vi "Read Config File.vi"(8 "error in (no error)":errorcluster, 11 "Config In":refnum<class "Excel_class.lvclass">=refnum) -> (0 "error out":errorcluster, 2 "Calibration Configuration Out":T1, 3 "DAQmx Cluster Out":T2 {"ai DAQmx Cluster"."input terminal configuration" items=["Default"=-1, "RSE"=10083, "NRSE"=10078, "Differential"=10106, "Pseudodifferential"=12529]; "bc DAQmx Cluster"."Scaling Information"."electrical units" items=["Volts/Volt"=15896, "mVolts/Volt"=15897]; "bc DAQmx Cluster"."Scaling Information"."physical units" items=["Newtons"=15875, "Pounds"=15876, "kgf"=15877]; "bc DAQmx Cluster"."Bridge Information"."bridge configuration" items=["Full Bridge"=10182, "Half Bridge"=10187, "Quarter Bridge"=10270]; "bc DAQmx Cluster"."Bridge Information"."voltage excitation source" items=["Internal"=10200, "External"=10167]; "tc DAQmx Cluster"."Thermocouple Type" items=["J"=10072, "K"=10073, "N"=10077, "R"=10082, "S"=10085, "T"=10086, "B"=10047, "E"=10055]; "tc DAQmx Cluster"."Units" items=["Deg C"=10143, "Deg F"=10144, "Kelvins"=10325, "Deg R"=10145, "From Custom Scale"=10065]})   [LabVIEW 2024]
uses:
  Calibration Configuration.ctl
  DAQmx Configuration.ctl
  <vilib>/ATEsystem/CLAUDIE_xlsx/Excel_class/Excel_class.lvclass
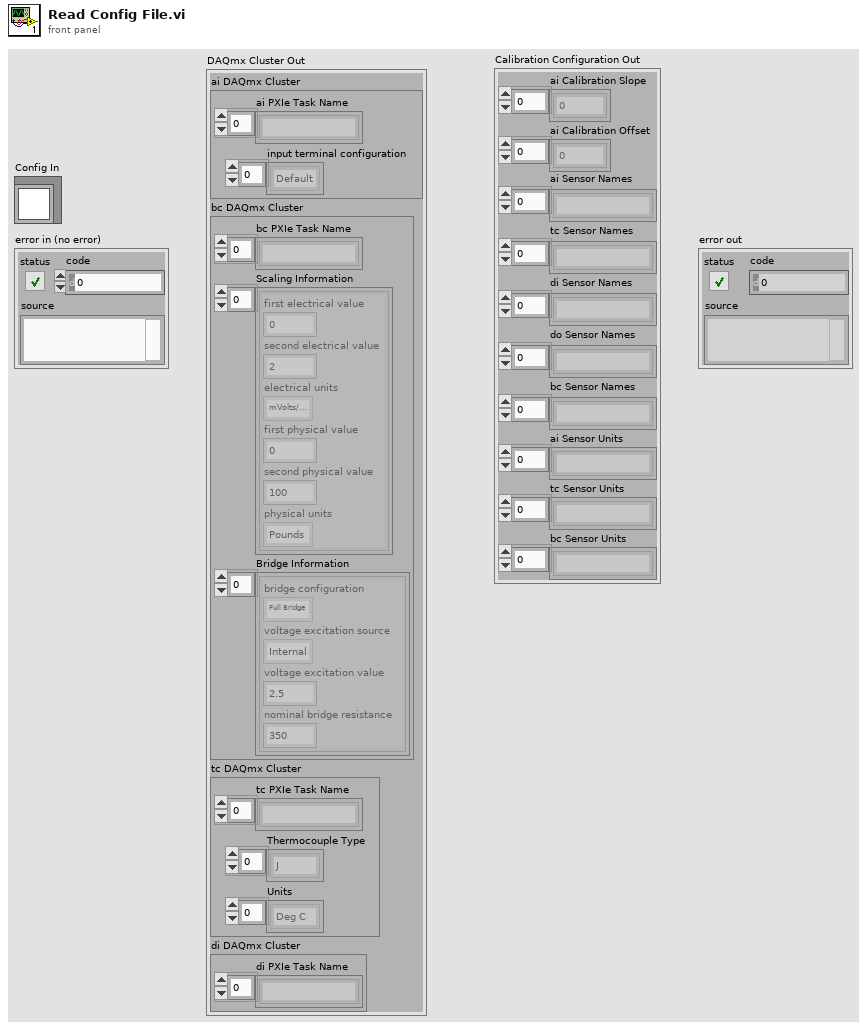
[diagram p1: front panel]
types:
  T1 = typedef "Calibration Configuration.ctl" = cluster{"ai Calibration Slope":dbl[], "ai Calibration Offset":dbl[], "ai Sensor Names ":string[], "tc Sensor Names":string[], "di Sensor Names":string[], "do Sensor Names":string[], "bc Sensor Names":string[], "ai Sensor Units":string[], "tc Sensor Units":string[], "bc Sensor Units":string[]}
  T2 = typedef "DAQmx Configuration.ctl" = cluster{"ai DAQmx Cluster":cluster{"ai PXIe Task Name":string[], "input terminal configuration":i32[]}, "bc DAQmx Cluster":cluster{"bc PXIe Task Name":string[], "Scaling Information":cluster{"first electrical value":dbl, "second electrical value":dbl, "electrical units":i32, "first physical value":dbl, "second physical value":dbl, "physical units":i32}[], "Bridge Information":cluster{"bridge configuration":i32, "voltage excitation source":i32, "voltage excitation value":dbl, "nominal bridge resistance":dbl}[]}, "tc DAQmx Cluster":cluster{"tc PXIe Task Name":string[], "Thermocouple Type":i32[], "Units":i32[]}, "di DAQmx Cluster":cluster{"di PXIe Task Name":string[]}}
  T3 = cluster{"ai PXIe Task Name":string[], "input terminal configuration":i32[]}
  T4 = cluster{"bc PXIe Task Name":string[], "Scaling Information":cluster{"first electrical value":dbl, "second electrical value":dbl, "electrical units":i32, "first physical value":dbl, "second physical value":dbl, "physical units":i32}[], "Bridge Information":cluster{"bridge configuration":i32, "voltage excitation source":i32, "voltage excitation value":dbl, "nominal bridge resistance":dbl}[]}
  T5 = cluster{"tc PXIe Task Name":string[], "Thermocouple Type":i32[], "Units":i32[]}
  T6 = cluster{dbl, dbl, "electrical units":i32, dbl, dbl, "physical units":i32}
  T7 = cluster{"bridge configuration":i32, "voltage excitation source":i32, dbl, dbl}
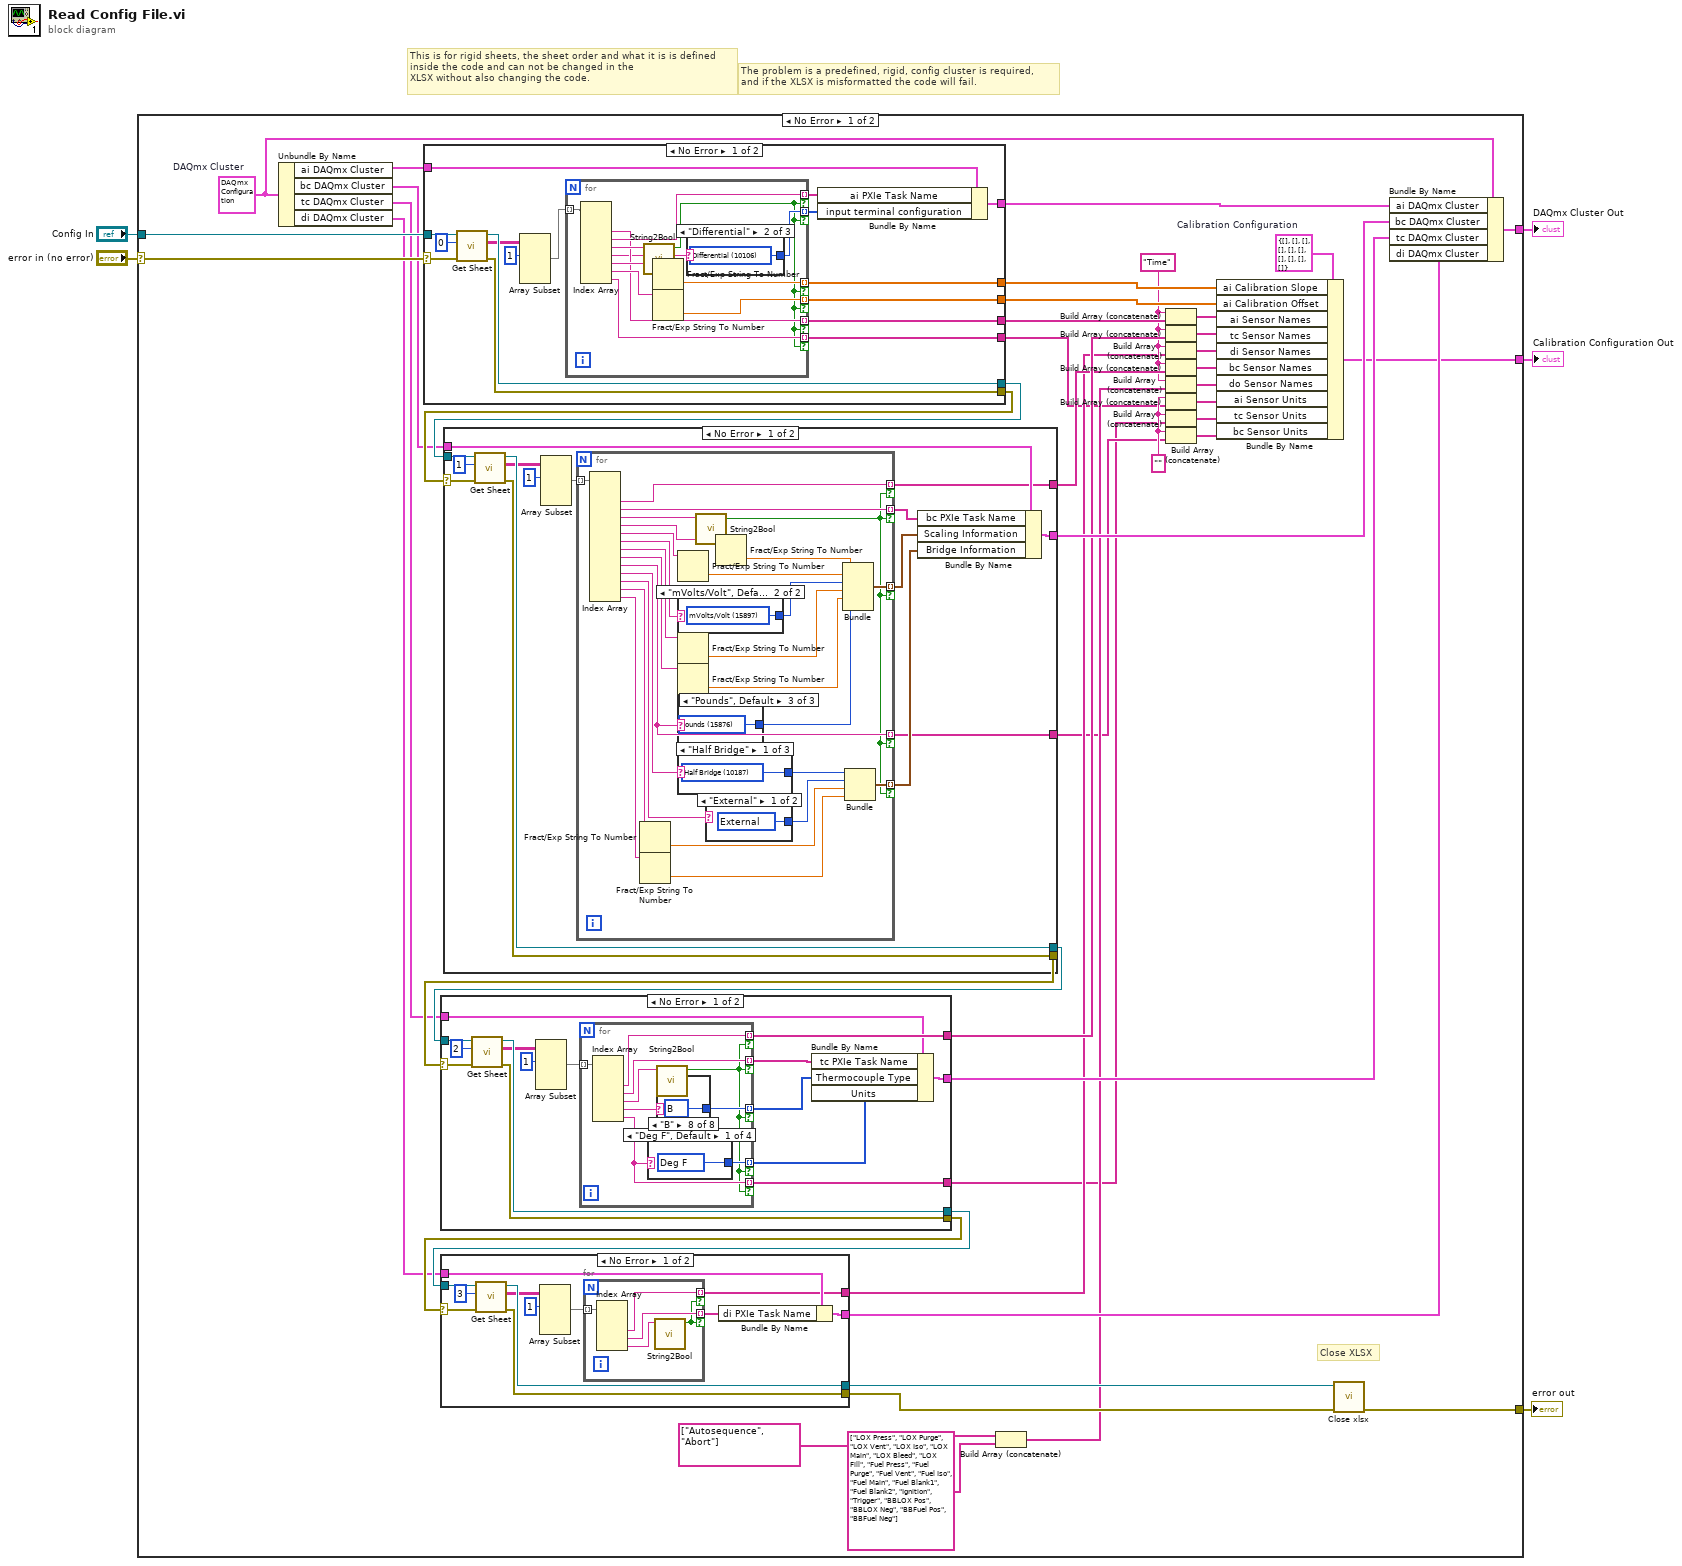
[diagram p0: block diagram]
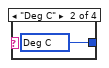
[diagram p3: hidden frame]
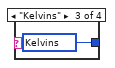
[diagram p4: hidden frame]
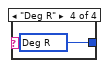
[diagram p5: hidden frame]
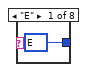
[diagram p6: hidden frame]
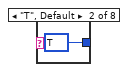
[diagram p7: hidden frame]
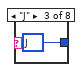
[diagram p8: hidden frame]
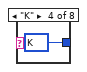
[diagram p9: hidden frame]
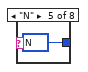
[diagram p10: hidden frame]
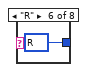
[diagram p11: hidden frame]
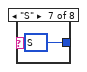
[diagram p12: hidden frame]
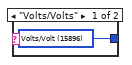
[diagram p14: hidden frame]
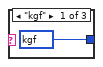
[diagram p15: hidden frame]
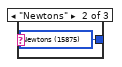
[diagram p16: hidden frame]
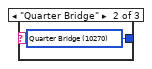
[diagram p17: hidden frame]
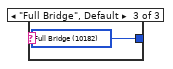
[diagram p18: hidden frame]
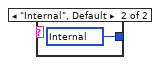
[diagram p19: hidden frame]
diagram:
  # "The problem is a predefined, rigid, config cluster is required,\nand if the XLSX is misformatted the code will fail."
  # "This is for rigid sheets, the sheet order and what it is is defined\ninside the code and can not be changed in the\nXLSX without also changing the code."
  n1 = case shown="No Error" "error in (no error)" {
    selector: "error in (no error)" -> [w37 w196]
    tunnel: [w50 w196] -> w4
    tunnel: [w43 _] -> w2
    tunnel: "Config In" -> [w38 _]
    tunnel: [w26 _] -> w1
    frame No Error {
      w11 = ""
      w17 = "Time"
      w32 = T1 {"ai Calibration Slope"=[], "ai Calibration Offset"=[], "ai Sensor Names "=[], "tc Sensor Names"=[], "di Sensor Names"=[], "do Sensor Names"=[], "bc Sensor Names"=[], "ai Sensor Units"=[], "tc Sensor Units"=[], "bc Sensor Units"=[]}  # Calibration Configuration
      w36 = T2 {"ai DAQmx Cluster"={"ai PXIe Task Name"=[], "input terminal configuration"=[]}, "bc DAQmx Cluster"={"bc PXIe Task Name"=[], "Scaling Information"=[], "Bridge Information"=[]}, "tc DAQmx Cluster"={"tc PXIe Task Name"=[], "Thermocouple Type"=[], "Units"=[]}, "di DAQmx Cluster"={"di PXIe Task Name"=[]}}  # DAQmx Cluster
      # "Close XLSX"
      n2 = Unbundle By Name(w36) -> ("ai DAQmx Cluster"=w48:T3, "bc DAQmx Cluster"=w35:T4, "tc DAQmx Cluster"=w34:T5, "di DAQmx Cluster"=w33:cluster{"di PXIe Task Name":string[]})
      n3 = case shown="No Error" w37 {
        selector: w37 -> [w175 w195]
        tunnel: w38 -> [w176 w194]
        tunnel: [w174 w193] -> w49
        tunnel: w48 -> [w173 w193]
        tunnel: [w172 w195] -> w47
        tunnel: [w171 w194] -> w46
        tunnel: [w165 _] -> w31
        tunnel: [w164 _] -> w30
        tunnel: [w163 _] -> w21
        tunnel: [w162 _] -> w8
        frame No Error {
          n4 = call <vilib>:"Get Sheet.vi"("error in (no error)"=w175, "List_index"=0, "Excel_class"=w176) -> ("error out"=w172:errorcluster, "Shared_strings"=w170:string[][], "Excel_class"=w171:refnum<class "Excel_class.lvclass">)  [unwired: 5 in, 1 out]
          n5 = Array Subset(array=w170, index (row)=1 ("index")) -> (w169:string[][])  [unwired: 3 in]
          n6 = for {
            tunnel: w169 -> [w189] mode=indexing
            tunnel: [w185] -> w167 mode=indexing if=w178
            tunnel: [w180] -> w166 mode=indexing if=w178
            tunnel: [w184] -> w165 mode=indexing if=w178
            tunnel: [w183] -> w164 mode=indexing if=w178
            tunnel: [w182] -> w163 mode=indexing if=w178
            tunnel: [w179] -> w162 mode=indexing if=w178
            n7 = Index Array(array=w189) -> (element #2=w182:string, element #3=w185:string, element #4=w188:string, element #5=w181:string, element #6=w187:string, element #7=w186:string, element #8=w179:string)  [unwired: 8 in, 1 out]
            n8 = call "String2Bool.vi"("String"=w188) -> ("Boolean"=w178:bool)  [unwired: 6 in]
            n9 = Fract/Exp String To Number(string=w187) -> (number=w184:dbl)  [unwired: 3 in, 1 out]
            n10 = Fract/Exp String To Number(string=w186) -> (number=w183:dbl)  [unwired: 3 in, 1 out]
            n11 = case shown="\"Differential\"" w181 {
              tunnel: [w190 w191 w192] -> w180
              frame "Default", Default {
                w190 = -1 items=["Default"=-1, "RSE"=10083, "NRSE"=10078, "Differential"=10106, "Pseudodifferential"=12529] ("input terminal configuration")
              }
              frame "Differential" {
                w191 = 10106 items=["Default"=-1, "RSE"=10083, "NRSE"=10078, "Differential"=10106, "Pseudodifferential"=12529] ("input terminal configuration")
              }
              frame "NRSE" {
                w192 = 10078 items=["Default"=-1, "RSE"=10083, "NRSE"=10078, "Differential"=10106, "Pseudodifferential"=12529] ("input terminal configuration")
              }
            }
          }
          n12 = Bundle By Name(cluster=w173, "ai PXIe Task Name"=w167, "input terminal configuration"=w166) -> (w174:T3)
        }
        frame Error {
        }
      }
      n13 = case shown="No Error" w47 {
        selector: w47 -> [w120 w161]
        tunnel: w46 -> [w121 w160]
        tunnel: [w119 w161] -> w45
        tunnel: [w118 w160] -> w44
        tunnel: w35 -> [w114 _]
        tunnel: [w111 _] -> w19
        tunnel: [w109 _] -> w29
        tunnel: [w108 _] -> w7
        frame No Error {
          n14 = call <vilib>:"Get Sheet.vi"("error in (no error)"=w120, "List_index"=1, "Excel_class"=w121) -> ("error out"=w119:errorcluster, "Shared_strings"=w117:string[][], "Excel_class"=w118:refnum<class "Excel_class.lvclass">)  [unwired: 5 in, 1 out]
          n15 = Array Subset(array=w117, index (row)=1 ("index")) -> (w115:string[][])  [unwired: 3 in]
          n16 = for {
            tunnel: w115 -> [w149] mode=indexing
            tunnel: [w141] -> w113 mode=indexing if=w123
            tunnel: [w136] -> w112 mode=indexing if=w123
            tunnel: [w135] -> w111 mode=indexing if=w123
            tunnel: [w134] -> w110 mode=indexing if=w123
            tunnel: [w124] -> w108 mode=indexing if=w123
            n17 = Index Array(array=w149) -> (element #2=w135:string, element #3=w136:string, element #4=w143:string, element #5=w148:string, element #6=w147:string, element #7=w128:string, element #8=w146:string, element #9=w145:string, element #10=w124:string, element #11=w131:string, element #12=w132:string, element #13=w144:string, element #14=w126:string)  [unwired: 14 in, 1 out]
            n18 = Fract/Exp String To Number(string=w144) -> (number=w142:dbl)  [unwired: 3 in, 1 out]
            n19 = Fract/Exp String To Number(string=w126) -> (number=w125:dbl)  [unwired: 3 in, 1 out]
            n20 = Fract/Exp String To Number(string=w147) -> (number=w139:dbl)  [unwired: 3 in, 1 out]
            n21 = case shown="\"mVolts/Volt\", Default" w128 {
              tunnel: [w150 w151] -> w127
              frame "Volts/Volts" {
                w150 = 15896 items=["Volts/Volt"=15896, "mVolts/Volt"=15897] ("electrical units")
              }
              frame "mVolts/Volt", Default {
                w151 = 15897 items=["Volts/Volt"=15896, "mVolts/Volt"=15897] ("electrical units")
              }
            }
            n22 = Fract/Exp String To Number(string=w146) -> (number=w138:dbl)  [unwired: 3 in, 1 out]
            n23 = Fract/Exp String To Number(string=w145) -> (number=w137:dbl)  [unwired: 3 in, 1 out]
            n24 = case shown="\"Pounds\", Default" w124 {
              tunnel: [w152 w153 w154] -> w129
              frame "kgf" {
                w152 = 15877 items=["Newtons"=15875, "Pounds"=15876, "kgf"=15877] ("physical units")
              }
              frame "Newtons" {
                w153 = 15875 items=["Newtons"=15875, "Pounds"=15876, "kgf"=15877] ("physical units")
              }
              frame "Pounds", Default {
                w154 = 15876 items=["Newtons"=15875, "Pounds"=15876, "kgf"=15877] ("physical units")
              }
            }
            n25 = case shown="\"Half Bridge\"" w131 {
              tunnel: [w155 w156 w157] -> w130
              frame "Half Bridge" {
                w155 = 10187 items=["Full Bridge"=10182, "Half Bridge"=10187, "Quarter Bridge"=10270] ("bridge configuration")
              }
              frame "Quarter Bridge" {
                w156 = 10270 items=["Full Bridge"=10182, "Half Bridge"=10187, "Quarter Bridge"=10270] ("bridge configuration")
              }
              frame "Full Bridge", Default {
                w157 = 10182 items=["Full Bridge"=10182, "Half Bridge"=10187, "Quarter Bridge"=10270] ("bridge configuration")
              }
            }
            n26 = call "String2Bool.vi"("String"=w143) -> ("Boolean"=w123:bool)  [unwired: 6 in]
            n27 = case shown="\"External\"" w132 {
              tunnel: [w158 w159] -> w133
              frame "External" {
                w158 = 10167 items=["Internal"=10200, "External"=10167] ("voltage excitation source")
              }
              frame "Internal", Default {
                w159 = 10200 items=["Internal"=10200, "External"=10167] ("voltage excitation source")
              }
            }
            n28 = Fract/Exp String To Number(string=w148) -> (number=w140:dbl)  [unwired: 3 in, 1 out]
            n29 = Bundle(w140, w139, "electrical units"=w127, w138, w137, "physical units"=w129) -> (w134:T6)  [unwired: 1 in]
            n30 = Bundle("bridge configuration"=w130, "voltage excitation source"=w133, w142, w125) -> (w141:T7)  [unwired: 1 in]
          }
          n31 = Bundle By Name(cluster=w114, "bc PXIe Task Name"=w112, "Scaling Information"=w110, "Bridge Information"=w113) -> (w109:T4)
        }
        frame Error {
        }
      }
      n32 = case shown="No Error" w45 {
        selector: w45 -> [w82 w107]
        tunnel: w44 -> [w83 w106]
        tunnel: w34 -> [w75 _]
        tunnel: [w81 w107] -> w42
        tunnel: [w80 w106] -> w41
        tunnel: [w76 _] -> w23
        tunnel: [w71 _] -> w28
        tunnel: [w70 _] -> w6
        frame No Error {
          n33 = call <vilib>:"Get Sheet.vi"("error in (no error)"=w82, "List_index"=2, "Excel_class"=w83) -> ("error out"=w81:errorcluster, "Shared_strings"=w78:string[][], "Excel_class"=w80:refnum<class "Excel_class.lvclass">)  [unwired: 5 in, 1 out]
          n34 = Array Subset(array=w78, index (row)=1 ("index")) -> (w77:string[][])  [unwired: 3 in]
          n35 = for {
            tunnel: w77 -> [w93] mode=indexing
            tunnel: [w91] -> w76 mode=indexing if=w85
            tunnel: [w90] -> w74 mode=indexing if=w85
            tunnel: [w87] -> w72 mode=indexing if=w85
            tunnel: [w88] -> w73 mode=indexing if=w85
            tunnel: [w86] -> w70 mode=indexing if=w85
            n36 = Index Array(array=w93) -> (element #2=w91:string, element #3=w90:string, element #4=w92:string, element #5=w89:string, element #6=w86:string)  [unwired: 6 in, 1 out]
            n37 = case shown="\"Deg F\", Default" w86 {
              tunnel: [w94 w95 w96 w97] -> w87
              frame "Deg F", Default {
                w94 = 10144 items=["Deg C"=10143, "Deg F"=10144, "Kelvins"=10325, "Deg R"=10145, "From Custom Scale"=10065] ("units")
              }
              frame "Deg C" {
                w95 = 10143 items=["Deg C"=10143, "Deg F"=10144, "Kelvins"=10325, "Deg R"=10145, "From Custom Scale"=10065] ("units")
              }
              frame "Kelvins" {
                w96 = 10325 items=["Deg C"=10143, "Deg F"=10144, "Kelvins"=10325, "Deg R"=10145, "From Custom Scale"=10065] ("units")
              }
              frame "Deg R" {
                w97 = 10145 items=["Deg C"=10143, "Deg F"=10144, "Kelvins"=10325, "Deg R"=10145, "From Custom Scale"=10065] ("units")
              }
            }
            n38 = call "String2Bool.vi"("String"=w92) -> ("Boolean"=w85:bool)  [unwired: 6 in]
            n39 = case shown="\"B\"" w89 {
              tunnel: [w98 w99 w100 w101 w102 w103 w104 w105] -> w88
              frame "E" {
                w98 = 10055 items=["J"=10072, "K"=10073, "N"=10077, "R"=10082, "S"=10085, "T"=10086, "B"=10047, "E"=10055] ("thermocouple type")
              }
              frame "T", Default {
                w99 = 10086 items=["J"=10072, "K"=10073, "N"=10077, "R"=10082, "S"=10085, "T"=10086, "B"=10047, "E"=10055] ("thermocouple type")
              }
              frame "J" {
                w100 = 10072 items=["J"=10072, "K"=10073, "N"=10077, "R"=10082, "S"=10085, "T"=10086, "B"=10047, "E"=10055] ("thermocouple type")
              }
              frame "K" {
                w101 = 10073 items=["J"=10072, "K"=10073, "N"=10077, "R"=10082, "S"=10085, "T"=10086, "B"=10047, "E"=10055] ("thermocouple type")
              }
              frame "N" {
                w102 = 10077 items=["J"=10072, "K"=10073, "N"=10077, "R"=10082, "S"=10085, "T"=10086, "B"=10047, "E"=10055] ("thermocouple type")
              }
              frame "R" {
                w103 = 10082 items=["J"=10072, "K"=10073, "N"=10077, "R"=10082, "S"=10085, "T"=10086, "B"=10047, "E"=10055] ("thermocouple type")
              }
              frame "S" {
                w104 = 10085 items=["J"=10072, "K"=10073, "N"=10077, "R"=10082, "S"=10085, "T"=10086, "B"=10047, "E"=10055] ("thermocouple type")
              }
              frame "B" {
                w105 = 10047 items=["J"=10072, "K"=10073, "N"=10077, "R"=10082, "S"=10085, "T"=10086, "B"=10047, "E"=10055] ("thermocouple type")
              }
            }
          }
          n40 = Bundle By Name(cluster=w75, "tc PXIe Task Name"=w74, "Thermocouple Type"=w73, "Units"=w72) -> (w71:T5)
        }
        frame Error {
        }
      }
      n41 = case shown="No Error" w42 {
        selector: w42 -> [w60 w69]
        tunnel: w41 -> [w61 w68]
        tunnel: w33 -> [w54 _]
        tunnel: [w59 w69] -> w40
        tunnel: [w58 w68] -> w39
        tunnel: [w53 _] -> w14
        tunnel: [w51 _] -> w27
        frame No Error {
          n42 = call <vilib>:"Get Sheet.vi"("error in (no error)"=w60, "List_index"=3, "Excel_class"=w61) -> ("error out"=w59:errorcluster, "Shared_strings"=w56:string[][], "Excel_class"=w58:refnum<class "Excel_class.lvclass">)  [unwired: 5 in, 1 out]
          n43 = Array Subset(array=w56, index (row)=1 ("index")) -> (w55:string[][])  [unwired: 3 in]
          n44 = for {
            tunnel: w55 -> [w67] mode=indexing
            tunnel: [w65] -> w52 mode=indexing if=w63
            tunnel: [w64] -> w53 mode=indexing if=w63
            n45 = Index Array(array=w67) -> (element #2=w64:string, element #3=w65:string, element #4=w66:string)  [unwired: 4 in, 1 out]
            n46 = call "String2Bool.vi"("String"=w66) -> ("Boolean"=w63:bool)  [unwired: 6 in]
          }
          n47 = Bundle By Name(cluster=w54, "di PXIe Task Name"=w52) -> (w51:cluster{"di PXIe Task Name":string[]})
        }
        frame Error {
        }
      }
      n48 = Build Array (concatenate)(string[] ["Autosequence", "Abort"], string[] ["LOX Press", "LOX Purge", "LOX Vent", "LOX Iso", "LOX Main", "LOX Bleed", "LOX Fill", "Fuel Press", "Fuel Purge", "Fuel Vent", "Fuel Iso", "Fuel Main", "Fuel Blank1", "Fuel Blank2", "Ignition", "Trigger", "BBLOX Pos", "BBLOX Neg", "BBFuel Pos", "BBFuel Neg"]) -> (w15:string[])
      n49 = Build Array (concatenate)(w17, w21) -> (w25:string[])
      n50 = Build Array (concatenate)(w17, w23) -> (w24:string[])
      n51 = Build Array (concatenate)(w17, w14) -> (w22:string[])
      n52 = Build Array (concatenate)(w17, w19) -> (w20:string[])
      n53 = Build Array (concatenate)(w17, w15) -> (w18:string[])
      n54 = Build Array (concatenate)(w11, w8) -> (w10:string[])
      n55 = Build Array (concatenate)(w11, w6) -> (w9:string[])
      n56 = Build Array (concatenate)(w11, w7) -> (w12:string[])
      n57 = Bundle By Name(cluster=w32, "ai Calibration Slope"=w31, "ai Calibration Offset"=w30, "ai Sensor Names"=w25, "tc Sensor Names"=w24, "di Sensor Names"=w22, "bc Sensor Names"=w20, "do Sensor Names"=w18, "ai Sensor Units"=w10, "tc Sensor Units"=w9, "bc Sensor Units"=w12) -> (w26:T1)
      n58 = call <vilib>:"Close xlsx.vi"("error in (no error)"=w40, "Excel_class"=w39) -> ("error out"=w50:errorcluster)  [unwired: 9 in]
      n59 = Bundle By Name(cluster=w36, "ai DAQmx Cluster"=w49, "bc DAQmx Cluster"=w29, "tc DAQmx Cluster"=w28, "di DAQmx Cluster"=w27) -> (w43:T2)
    }
    frame Error {
    }
  }
  "error out" <- w4
  "DAQmx Cluster Out" <- w2
  "Calibration Configuration Out" <- w1
